vi "PC_Aquire_Still_Image (DONE).vi"(3 "Error In":errorcluster, 4 "Image In":T2, 5 "Session In":T1) -> (0 "Error Out":errorcluster, 1 "Image Out":T2(plugin-control), 2 "Session Out":T1)   [LabVIEW 2017]
uses:
  <vilib>/userdefined/High Color/IMAQdx.ctl
  <vilib>/vision/Image Controls.llb/IMAQ Image.ctl
  <vilib>/vision/driver/NI_Vision_Acquisition_Software.lvlib
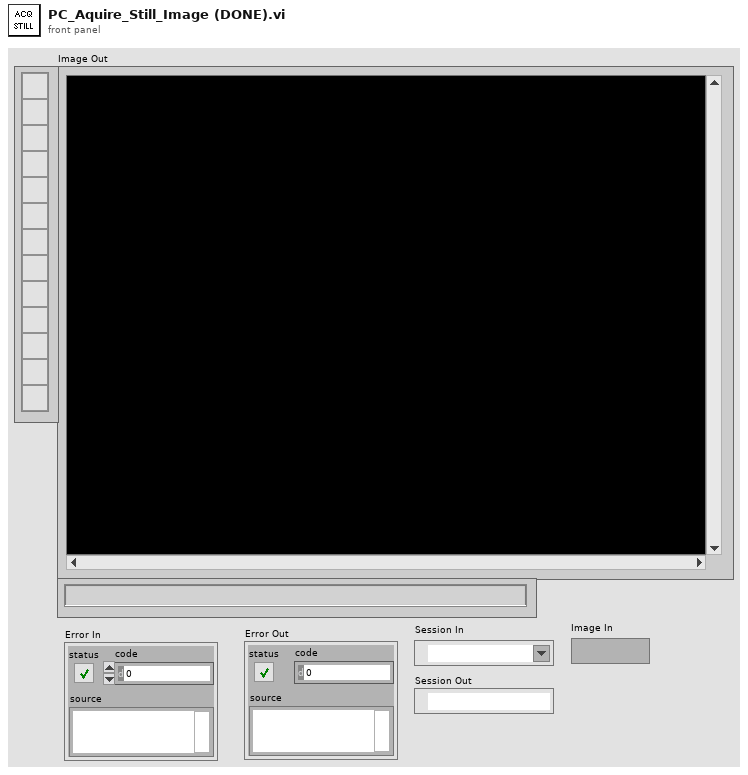
[diagram p1: front panel]
types:
  T1 = typedef "IMAQdx.ctl" = refnum<k21>
  T2 = typedef "IMAQ Image.ctl" = refnum<image>
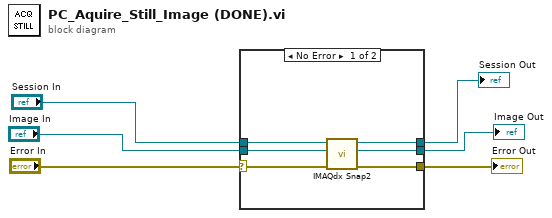
[diagram p0: block diagram]
diagram:
  n1 = case shown="No Error" "Error In" {
    selector: "Error In" -> [w11 w13]
    tunnel: [w10 w13] -> w6
    tunnel: [w12 w14] -> w5
    tunnel: "Session In" -> [w9 w15]
    tunnel: "Image In" -> [w8 w14]
    tunnel: [w7 w15] -> w1
    frame No Error {
      n2 = call <vilib>:"IMAQdx Snap2.vi"("error in"=w11, "Image In"=w8, "Session In"=w9) -> ("error out"=w10:errorcluster, "Image Out"=w12:T2, "Session Out"=w7:T1)  [unwired: 6 in]
    }
    frame Error {
    }
  }
  "Error Out" <- w6
  "Image Out" <- w5
  "Session Out" <- w1
